vi "Get Group and Channel Names From Tag.vi"(4 "error in":errorcluster, 7 "tree path":string) -> (0 "error out":errorcluster, 2 "channel":string, 3 "group":string)   [LabVIEW 2020, in "NI_TDMS File Viewer.lvlib"]
uses:
  <vilib>/Utility/TDMS File Viewer/NI_TDMS File Viewer.lvlib
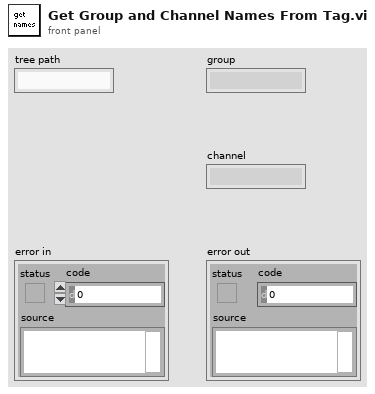
[diagram p1: front panel]
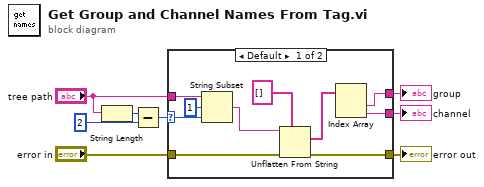
[diagram p0: block diagram]
diagram:
  n1 = String Length(string="tree path") -> (length=w4:i32)
  n2 = Subtract(x=w4, y=2 ("offset (0)")) -> (x-y=w1:i32)
  n3 = case shown="Default" w1 {
    selector: w1 -> [w14 _]
    tunnel: [w18 w19] -> w8
    tunnel: "error in" -> [w17 w19]
    tunnel: "tree path" -> [w16 _]
    tunnel: [w12 _] -> w3
    tunnel: [w11 _] -> w2
    frame Default {
      n4 = String Subset(string=w16, offset (0)=1, length (rest)=w14) -> (substring=w15:string)
      n5 = Unflatten From String(type=string[] [], binary string=w15, error in (no error)=w17) -> (value=w10:string[], error out=w18:errorcluster)  [unwired: 2 in, 1 out]
      n6 = Index Array(array=w10) -> (element #1=w11:string, element #2=w12:string)  [unwired: 2 in]
    }
    frame ..0 {
    }
  }
  "error out" <- w8
  "channel" <- w3
  "group" <- w2
